vi "Agilent SNA Set IFBW.vi"(6 "Channel":i8=1 min=1 max=99 step=1, 7 "Agilent SNA & SWP":T1, 8 "error in (no error)":errorcluster, 10 "IFBW, Hz (1000)":dbl=1000.0, 11 "VISA Resource Names":T2) -> (0 "error out":errorcluster, 3 "dup VISA Resource Names":T2)   [LabVIEW 2011]
doc: "This Vi for the HP8753B Network Analyzer is used to set averaging, smoothing, and the IF bandwidth."
uses:
  TypeDefs/Agilent SNA VISA.ctl
  TypeDefs/Agilent SNA Instrument Info.ctl
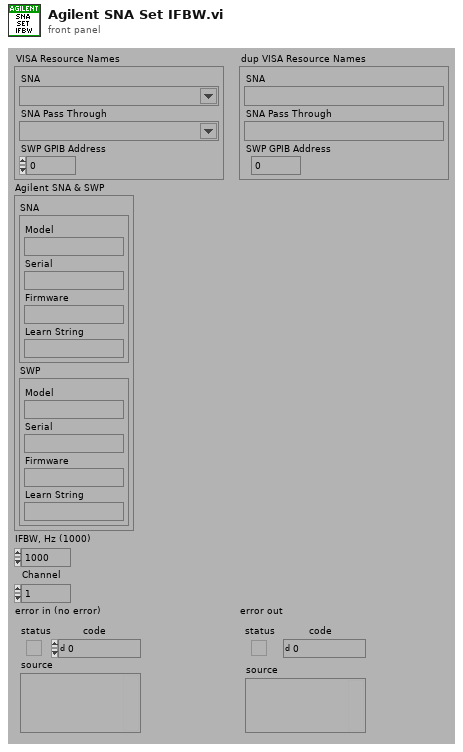
[diagram p1: front panel]
types:
  T1 = typedef "Agilent SNA Instrument Info.ctl" = cluster{"SNA":cluster{"Model":string, "Serial":string, "Firmware":string, "Learn String":string}, "SWP":cluster{"Model":string, "Serial":string, "Firmware":string, "Learn String":string}}
  T2 = typedef "Agilent SNA VISA.ctl" = cluster{"SNA":refnum<visa-resource-name>, "SNA Pass Through":refnum<visa-resource-name>, "SWP GPIB Address":i32}
  T3 = typedef "Agilent SNA Model.ctl" = enum16{"Not Supported", "8757X"}
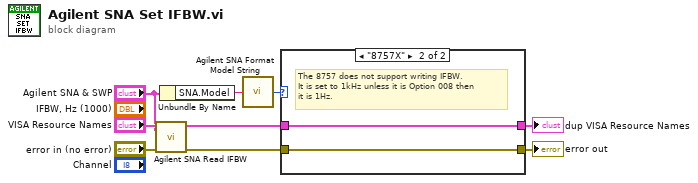
[diagram p0: block diagram]
diagram:
  n1 = call "Agilent SNA Read IFBW.vi"("Agilent SNA & SWP"="Agilent SNA & SWP", "error in (no error)"="error in (no error)", "VISA Resource Names"="VISA Resource Names") -> ("error out"=w6:errorcluster, "dup VISA Resource Name"=w2:T2)  [unwired: 1 in, 6 out]
  n2 = Unbundle By Name("Agilent SNA & SWP") -> ("SNA.Model"=w3:string)
  n3 = call "Agilent SNA Format Model String.vi"("Model String"=w3) -> ("Model"=w5:T3)
  n4 = case shown="\"8757X\"" w5 {
    tunnel: [w11 w13] -> w9
    tunnel: w6 -> [w11 w13]
    tunnel: w2 -> [w10 w12]
    tunnel: [w10 w12] -> w1
    frame "Not Supported" {
    }
    frame "8757X" {
      # "The 8757 does not support writing IFBW.\nIt is set to 1kHz unless it is Option 008 then\nit is 1Hz."
    }
  }
  "error out" <- w9
  "dup VISA Resource Names" <- w1
